vi "Cmd Get Command Properties (C).vi"(4 "error in (no error)":errorcluster, 7 "command reference":T2) -> (0 "error out":errorcluster, 1 "command properties":T1, 3 "command reference out":T2)   [LabVIEW 2013, in "NI_Database_API_64.lvlib"]
doc: "Gets properties of the object as determined by the inputs. This VI works for connections, commands, recordsets, columns, and parameters. Wire data to the reference input to determine the polymorphic instance to use or manually select the instance."
uses:
  NI_Database_API_64.lvlib
  Cmd ObjectReference.ctl
  Cmd Properties.ctl
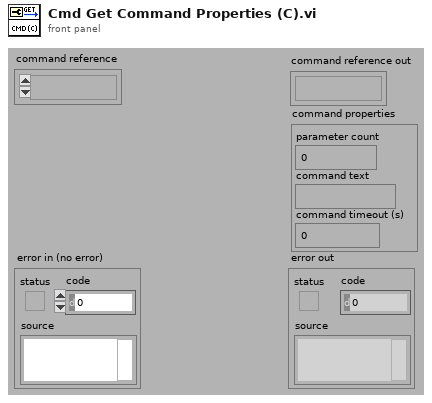
[diagram p1: front panel]
types:
  T1 = typedef "NI_Database_API_64.lvlib/Cmd Properties.ctl" = cluster{"parameter count":i32, "command text":string, "command timeout (s)":i32}
  T2 = typedef "NI_Database_API_64.lvlib/Cmd ObjectReference.ctl" = refnum<k1>
  T3 = cluster{"Count":i32, "CommandText":string, "CommandTimeout":i32}
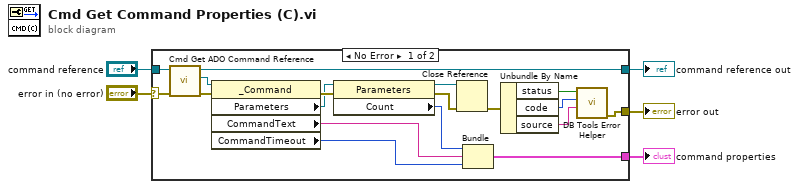
[diagram p0: block diagram]
diagram:
  n1 = case shown="No Error" "error in (no error)" {
    selector: "error in (no error)" -> [w6 w25]
    tunnel: [w16 _] -> w5
    tunnel: "command reference" -> [w13 w24]
    tunnel: [w12 w24] -> w3
    tunnel: [w7 w25] -> w2
    frame No Error {
      n2 = call "Cmd Get ADO Command Reference.vi"("error in (no error)"=w6, "command reference"=w13) -> ("error out"=w14:errorcluster, "ADODB._Command"=w15:refnum<k7>, "command reference out"=w12:T2)  [unwired: 3 out]
      n3 = property class="_Command"(reference=w15, error in=w14) -> (error out=w23:errorcluster, "Parameters"=w20:refnum<k7>, "CommandText"=w18:string, "CommandTimeout"=w17:i32)  [unwired: 1 out]
      n4 = property class="Parameters"(reference=w20, error in=w23) -> (reference out=w21:refnum<k7>, error out=w22:errorcluster, "Count"=w19:i32)
      n5 = Close Reference(reference=w21, error in (no error)=w22) -> (error out=w8:errorcluster)
      n6 = Bundle("Count"=w19, "CommandText"=w18, "CommandTimeout"=w17) -> (w16:T3)  [unwired: 1 out]
      n7 = Unbundle By Name(w8) -> ("status"=w10:bool, "code"=w9:i32, "source"=w11:string)
      n8 = call "DB Tools Error Helper.vi"("source"=w11, "code"=w9, "status"=w10) -> ("error out"=w7:errorcluster)  [unwired: 1 in, 7 out]
    }
    frame Error {
    }
  }
  "command reference out" <- w3
  "error out" <- w2
  "command properties" <- w5
